vi "Configure Auto Sweep Type.vi"(0 "VISA resource name":refnum<visa-resource-name>, 5 "Switching Rules (0:Dynamic Range)":i32(ring) items=["Dynamic Range", "Measurement Speed", "Only Sweep", "Priortize Sweep", "Prioritize FFT"], 7 "FFT Width (40000:40kHz)":dbl(ring)=40000.0 items=["40kHz"=40000.0, "2MHz"=2000000.0], 11 "error in (no error)":errorcluster) -> (4 "VISA resource name out":refnum<visa-resource-name>, 15 "error out":errorcluster)   [LabVIEW 2020, in "Anritsu Signal Analyzer Series.lvlib"]
doc: "Configures the auto sweep type and FFT width settings of the spectrum analyzer."
uses:
  Anritsu Signal Analyzer Series.lvlib
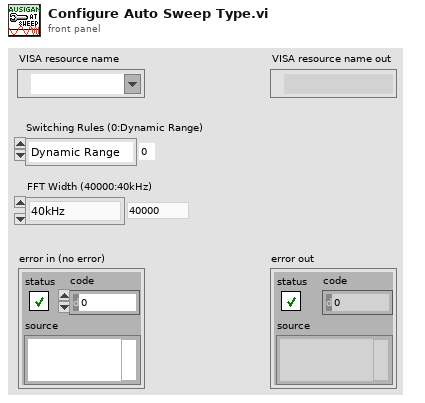
[diagram p1: front panel]
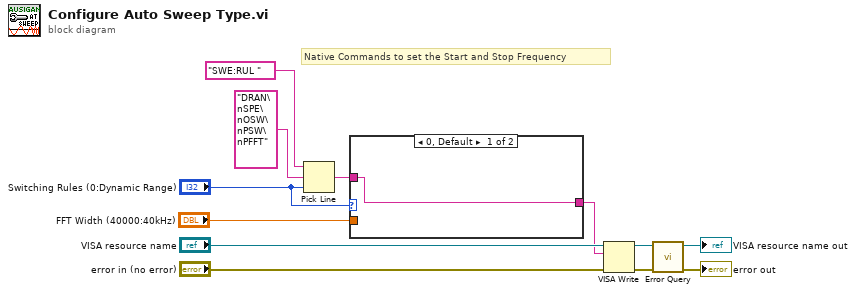
[diagram p0: block diagram]
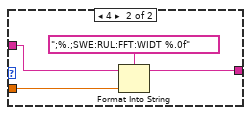
[diagram p2: hidden frame]
diagram:
  # "Native Commands to set the Start and Stop Frequency"
  n1 = Pick Line(string ("")="SWE:RUL " ("_Command Set"), multi-line string="DRAN\nSPE\nOSW\nPSW\nPFFT" ("複数行文字列"), line index="Switching Rules (0:Dynamic Range)") -> (output string=w4:string)
  n2 = case shown="0, Default" "Switching Rules (0:Dynamic Range)" {
    tunnel: w4 -> [w13 w16]
    tunnel: "FFT Width (40000:40kHz)" -> [_ w15]
    tunnel: [w13 w14] -> w1
    frame 0, Default {
    }
    frame 4 {
      n3 = Format Into String(format string=";%.;SWE:RUL:FFT:WIDT %.0f", initial string=w16, w15) -> (resulting string=w14:string)  [unwired: 1 in, 1 out]
    }
  }
  n4 = VISA Write(VISA resource name="VISA resource name", write buffer=w1, error in (no error)="error in (no error)") -> (VISA resource name out=w7:refnum<visa-resource-name>, error out=w8:errorcluster)  [unwired: 1 out]
  n5 = call "Error Query.vi"("error in (no error)"=w8, "VISA resource name"=w7) -> ("error out"=→"error out":errorcluster, "VISA resource name out"=→"VISA resource name out":refnum<visa-resource-name>)  [unwired: 6 in, 2 out]
